vi "Create_Dests.vi"(8 "error in (no error)":errorcluster, 11 "Class in":refnum<class "IB_MSI.lvclass">) -> (0 "error out":errorcluster, 3 "Class out":refnum<class "IB_MSI.lvclass">)   [LabVIEW 2020, in "IB_MSI.lvclass"]
uses:
  <vilib>/AppBuilder/IB_Classes/MSI/IB_MSI.lvclass
  <vilib>/AppBuilder/IB_Classes/MSI/IB_MSI.lvclass/IB_MSI.ctl
  <resource>/Framework/Providers/Builds/Installer/CDK_GLOBAL_LABELS.vi
  <vilib>/AppBuilder/IB_Classes/Destination/IB_Destination.lvclass
  <vilib>/AppBuilder/IB_Classes/Installer/Installer.lvclass
  <vilib>/AppBuilder/IB_Classes/Dest_NI_MSIPath/Dest_NI_MSIPath.lvclass
  e:/builds/penguin/labview/branches/2020/dev/dist/vi.lib/AppBuilder/IB_Classes/Installer/Installer.lvclass
  e:/builds/penguin/labview/branches/2020/dev/dist/vi.lib/AppBuilder/IB_Classes/MSI/IB_MSI.lvclass
  e:/builds/penguin/labview/branches/2020/dev/dist/vi.lib/AppBuilder/IB_Classes/Destination/niLabel/niLabel.lvclass
  e:/builds/penguin/labview/branches/2020/dev/dist/vi.lib/AppBuilder/IB_Classes/Destination/IB_Destination.lvclass
  e:/builds/penguin/labview/branches/2020/dev/dist/vi.lib/AppBuilder/IB_Classes/Dest_NI_MSIPath/Dest_NI_MSIPath.lvclass
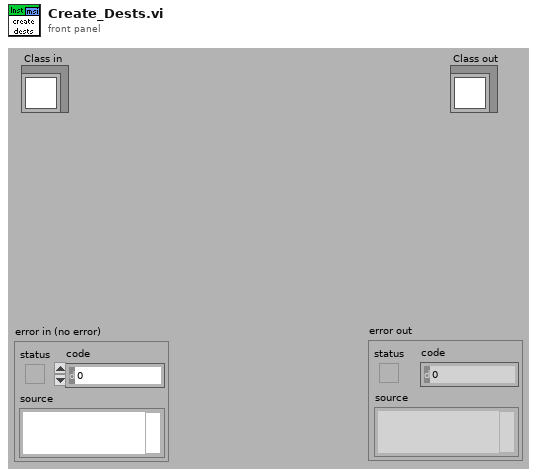
[diagram p1: front panel]
types:
  T1 = typedef "CDK_sTypeDef_AppBitness.ctl" = enum16{"invalid", "32-bit", "64-bit"}
  T2 = typedef "IB_Destination.ctl" = cluster{"name":string, "unlock":bool, "parentTag":string, "destTag":string, "eng_installPath":string}
  T3 = typedef "IB_Installer.ctl" = cluster{"Destination":refnum<class "IB_Destination.lvclass">[], "Source":refnum<class "IB_Source.lvclass">[], "buildObject":T4, "defaultDir":string, "platform":string, "author":string, "productName":string, "buildSpecName":string, "hide":bool, "requireLVDevSys":bool, "autoIncrement":bool, "includeError":bool, "readmeID":string, "buildLocation":path, "readmePath":path, "mediaSize":u16, "language":T5, "productVersion":T6, "preview":bool, "programmatic":bool, "progressBarEvents":T7, "userLog_Path":path, "shortcutAddresses":T9[], "EXE_Install Address":string, "EXE_Uninstall Address":string, "additional NIPaths":refnum<class "Dest_NI_NIPath.lvclass">[], "web service itemIDs":string[], "installerName":string}
  T4 = typedef "ItemRef.ctl" = u64
  T5 = typedef "CDK_sTypeDef_Languages.ctl" = u16
  T6 = typedef "CDK_sTypeDef_ProductVersion.ctl" = cluster{"Major":u8, "Minor":u8, "Update":u16}
  T7 = typedef "provcom_ProgressBar_Events.ctl" = cluster{"newJob":refnum<user-event>, "newItem":refnum<user-event>, "errorMsg":T8, "cancel":refnum<user-event>}
  T8 = typedef "mxLvBuildError.ctl" = refnum<user-event>
  T9 = typedef "CDK_sTypeDef_ShortcutAddress.ctl" = cluster{"file":string, "shortcut":string}
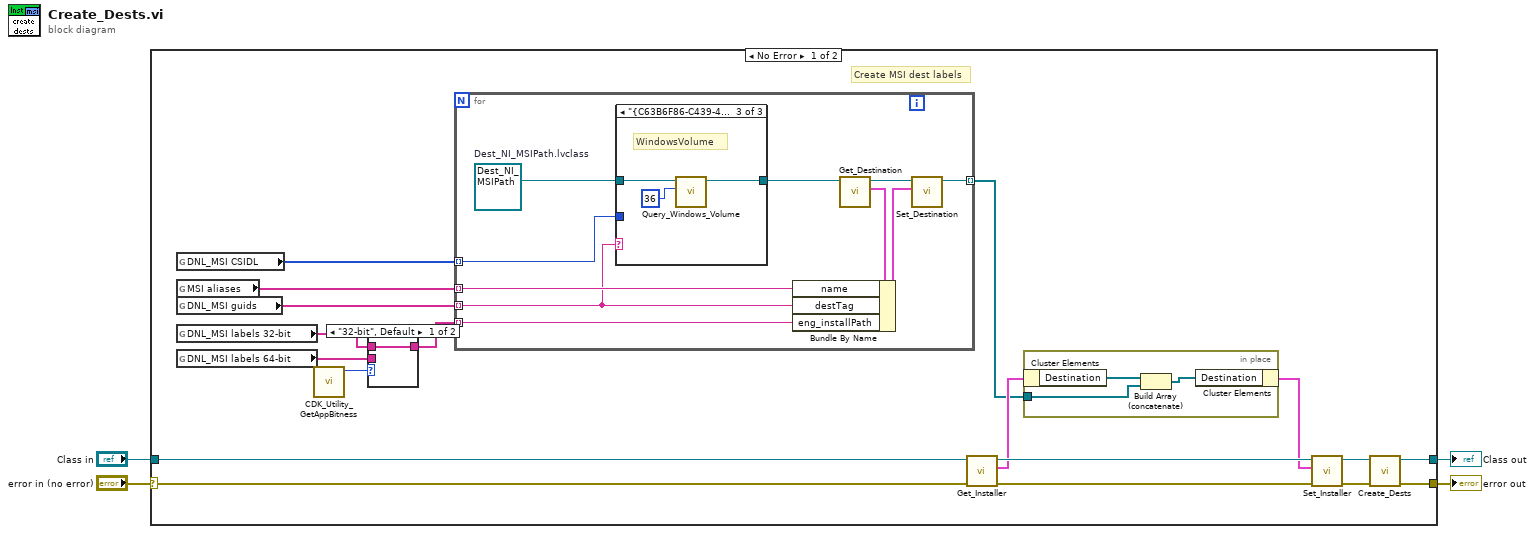
[diagram p0: block diagram]
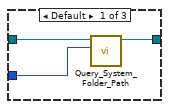
[diagram p3: hidden frame]
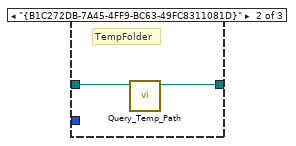
[diagram p4: hidden frame]
diagram:
  n1 = case shown="No Error" "error in (no error)" {
    selector: "error in (no error)" -> [w19 w46]
    tunnel: "Class in" -> [w22 w47]
    tunnel: [w17 w47] -> w3
    tunnel: [w15 w46] -> w1
    frame No Error {
      # "Create MSI dest labels"
      n2 = global read "CDK_GLOBAL_LABELS.vi" "DNL_MSI CSIDL"() -> (w5:u8[])
      n3 = global read "CDK_GLOBAL_LABELS.vi" "MSI aliases"() -> (w14:string[])
      n4 = global read "CDK_GLOBAL_LABELS.vi" "DNL_MSI guids"() -> (w13:string[])
      n5 = global read "CDK_GLOBAL_LABELS.vi" "DNL_MSI labels 32-bit"() -> (w8:string[])
      n6 = global read "CDK_GLOBAL_LABELS.vi" "DNL_MSI labels 64-bit"() -> (w7:string[])
      n7 = call <resource>:"CDK_Utility_GetAppBitness.vi"() -> ("app bitness"=w9:T1)  [unwired: 11 out]
      n8 = case shown="\"32-bit\", Default" w9 {
        tunnel: w7 -> [_ w24]
        tunnel: [w23 w24] -> w6
        tunnel: w8 -> [w23 _]
        frame "32-bit", Default {
        }
        frame "64-bit" {
        }
      }
      n9 = for {
        tunnel: w14 -> [w37] mode=indexing
        tunnel: [w33] -> w11 mode=indexing
        tunnel: w13 -> [w31] mode=indexing
        tunnel: w6 -> [w32] mode=indexing
        tunnel: w5 -> [w28] mode=indexing
        w30 = refnum<class "Dest_NI_MSIPath.lvclass"> refnum  # Dest_NI_MSIPath.lvclass
        n10 = case shown="\"{C63B6F86-C439-4240-9AAE-EC6A9DDD0A29}\"" w31 {
          tunnel: w30 -> [w40 w42 w45]
          tunnel: [w39 w41 w44] -> w29
          tunnel: w28 -> [w38 _ _]
          frame Default {
            n11 = call <vilib>:"Query_System_Folder_Path.vi"("nFolder"=w38, "Dest_NI_MSIPath in"=w40) -> ("Dest_NI_MSIPath out"=w39:refnum<class "Dest_NI_MSIPath.lvclass">)  [unwired: 7 in, 2 out]
          }
          frame "{B1C272DB-7A45-4FF9-BC63-49FC8311081D}" {
            # "TempFolder"
            n12 = call <vilib>:"Query_Temp_Path.vi"("Dest_NI_MSIPath in"=w42) -> ("Dest_NI_MSIPath out"=w41:refnum<class "Dest_NI_MSIPath.lvclass">)  [unwired: 9 in, 1 out]
          }
          frame "{C63B6F86-C439-4240-9AAE-EC6A9DDD0A29}" {
            # "WindowsVolume"
            n13 = call <vilib>:"Query_Windows_Volume.vi"("nFolder"=u8 36, "Dest_NI_MSIPath in"=w45) -> ("Dest_NI_MSIPath out"=w44:refnum<class "Dest_NI_MSIPath.lvclass">)  [unwired: 8 in, 1 out]
          }
        }
        n14 = call <vilib>:"Get_Destination.vi"("IB_Destination in"=w29) -> ("data"=w35:T2, "IB_Destination out"=w36:refnum<class "Dest_NI_MSIPath.lvclass">)  [unwired: 8 in, 1 out]
        n15 = Bundle By Name(cluster=w35, "name"=w37, "destTag"=w31, "eng_installPath"=w32) -> (w34:T2)
        n16 = call <vilib>:"Set_Destination.vi"("data"=w34, "IB_Destination in"=w36) -> ("IB_Destination out"=w33:refnum<class "Dest_NI_MSIPath.lvclass">)  [unwired: 8 in, 1 out]
      }
      n17 = call <vilib>:"Get_Installer.vi"("error in (no error)"=w19, "Installer in"=w22) -> ("error out"=w20:errorcluster, "data"=w12:T3, "Installer out"=w21:refnum<class "IB_MSI.lvclass">)  [unwired: 7 in]
      n18 = in-place {
        in-place-border: w11 -> [w26]
        n19 = in-place-cluster #1(w12) -> ("Destination"=w27:refnum<class "IB_Destination.lvclass">[])
        n20 = Build Array (concatenate)(w27, w26) -> (w25:refnum<class "IB_Destination.lvclass">[])
        n21 = in-place-cluster #1("Destination"=w25) -> (w10:T3)
      }
      n22 = call <vilib>:"Set_Installer.vi"("error in (no error)"=w20, "data"=w10, "Installer in"=w21) -> ("error out"=w16:errorcluster, "Installer out"=w18:refnum<class "IB_MSI.lvclass">)  [unwired: 7 in]
      n23 = call-parent "Create_Dests.vi"("error in (no error)"=w16, "Class in"=w18) -> ("error out"=w15:errorcluster, "Class out"=w17:refnum<class "IB_MSI.lvclass">)  [unwired: 8 out]
    }
    frame Error {
    }
  }
  "error out" <- w1
  "Class out" <- w3
